vi "LIDAR V5 FPGA Main.vi"() -> ()   [LabVIEW 2015]
uses:
  <vilib>/Platform/TimedLoop/XDataNode/XDataNode.xnode
  <vilib>/Platform/TimedLoop/XDataNode/nitl_modes.ctl
  <vilib>/Platform/TimedLoop/XDataNode/XDNodeRunTimeDep.lvlib
  <vilib>/Platform/TimedLoop/XDataNode/wakeup.ctl
  <vilib>/Platform/TimedLoop/XDataNode/timing_clust.ctl
  <vilib>/eio/EIONode/EIONode.xnode
  <vilib>/rvi/eio/common/nirviEmuTemplateMethod_errors.vi
  <vilib>/rvi/DataTransferAndStorage/Container/XNode/niFpgaContainer.xnode
  <vilib>/rvi/FIFO/Fifo_Resource/nirvififoEmulationRead.vi
  LIDAR V2 Globals.vi
  <vilib>/rvi/Memory/Memory_Emulation/nirvimemoryFastEmulation.vi
  <vilib>/rvi/Memory/Memory_Emulation/nirvimemoryEmulation.vi
  Controls/FPGA Nain State.ctl
  Controls/Algorithm State.ctl
  <vilib>/rvi/interface/RandomDataEmulation/nirviRandomDataFpgaReadWriteTemplate.vi
panel:
  in  "y 6":u32
  in  "y 5":u32
  out "PulseIndex":i16
  in  "WaitForPulseEndDelay":u8=3
  in  "y":i16
  in  "y 2":i16
  in  "y 3":i16
  in  "y 4":i16
  out "EnableSignal":bool
  out "ActiveLedIndex":u16
  in  "EndOfPulseGen 2":bool
  in  "SamplingEnable":bool
  in  "SingleFrame":bool
  out "MainState":T1
  in  "NoOfLeds":u16=320
  in  "PulsePerLed":i16=199
  in  "FillDark":bool
  in  "DarkData":fxp<+/-,22,22>
  in  "DarkAdd":u32
  in  "SubstractDark":bool
  in  "FillVga":bool
  in  "VgaData":i16
  in  "VgaAdd":u32
  in  "ScanMode":bool
  in  "FrameStartDisable":bool=TRUE
  out "MeanTimeouts":u16
  in  "MaxStartSample":u32
  out "Port1":u8 format="%.0b"
  out "Port1Bit5":bool
  out "Port1Bit4":bool
  out "Port0":u8 format="%.0b"
  in  "PFI2":bool
  in  "PFI3":bool
  in  "ActiveLedIndexDeb":u16
  in  "LedScanDebEn":bool
  out "User Command Idle":bool
  out "User Command Status":u8
  out "User Error":bool
  out "Configured?":bool
  out "PLL Locked":bool
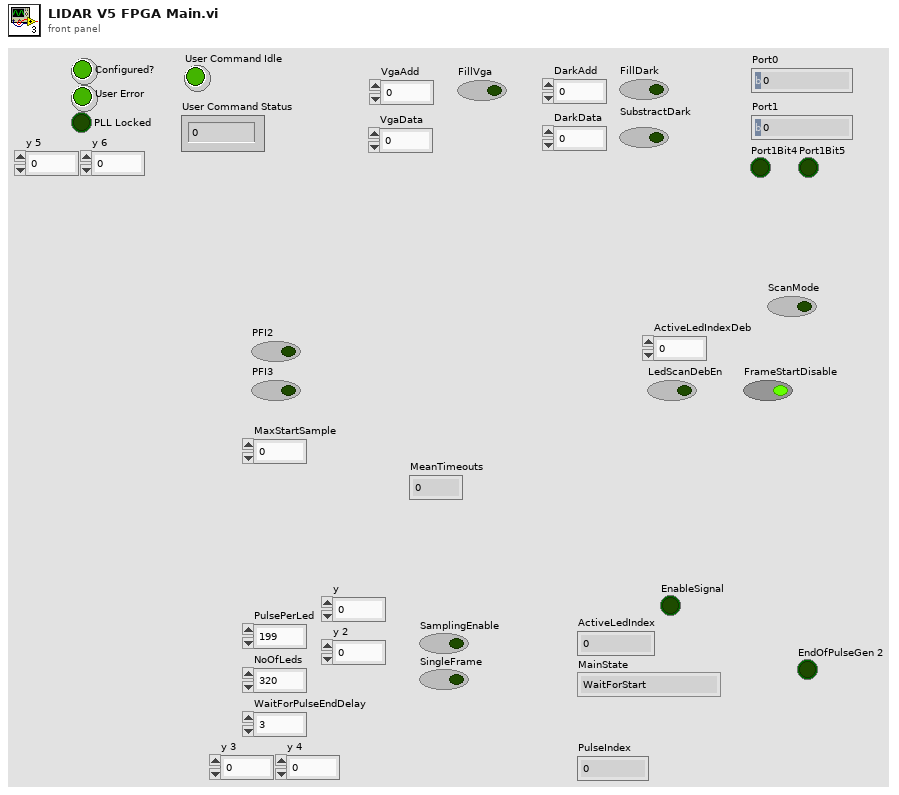
[diagram p1: front panel]
types:
  T1 = typedef "FPGA Nain State.ctl" = enum16{"WaitForStart", "SelectActiveLed", "WaitForNextPulse", "ActivatePulseCycle", "Error"}
  T2 = typedef "XDNodeRunTimeDep.lvlib/timing_clust.ctl" = cluster{"Expected End [f-1]":u64, "Actual End [f-1]":u64, "Finished Late? [f-1]":bool, "Expected End [i-1]":u64, "Actual End [i-1]":u64, "Finished Late? [i-1]":bool, "Expected Start [i]":u64, "Actual Start [i]":u64, "Expected Start [f]":u64, "Actual Start [f]":u64, "Source Name":string, "Structure Name":string, "Period":i64, "Deadline":i64, "Offset":i64, "Start":i64, "Priority":i32, "Timeout":i32, "Mode":T3, "Wakeup Reason":T4, "Error":errorcluster, "Source Type":string, "Secondary Source Type":string, "Global End Time":u64, "Global Start Time":u64, "Frame Duration":u64, "Iteration Duration":u64, "Assigned CPU":i32, "I/O Scan Engine Mode":u32}
  T3 = typedef "XDNodeRunTimeDep.lvlib/nitl_modes.ctl" = enum32{"No Change", "Process missed periods, maintain original phase", "Discard missed periods, maintain original phase", "Process missed periods, ignore original phase", "Discard missed periods, ignore original phase"}
  T4 = typedef "XDNodeRunTimeDep.lvlib/wakeup.ctl" = enum32{"Normal", "Aborted", "Asynchronous wakeup", "Timing source error", "Timed loop error", "Timeout"}
  T5 = typedef "Algorithm State.ctl" = enum16{"WaitForStart", "GetNextSignalElement", "WaitForNextSignalElem", "MultWithSinc", "CalcMax"}
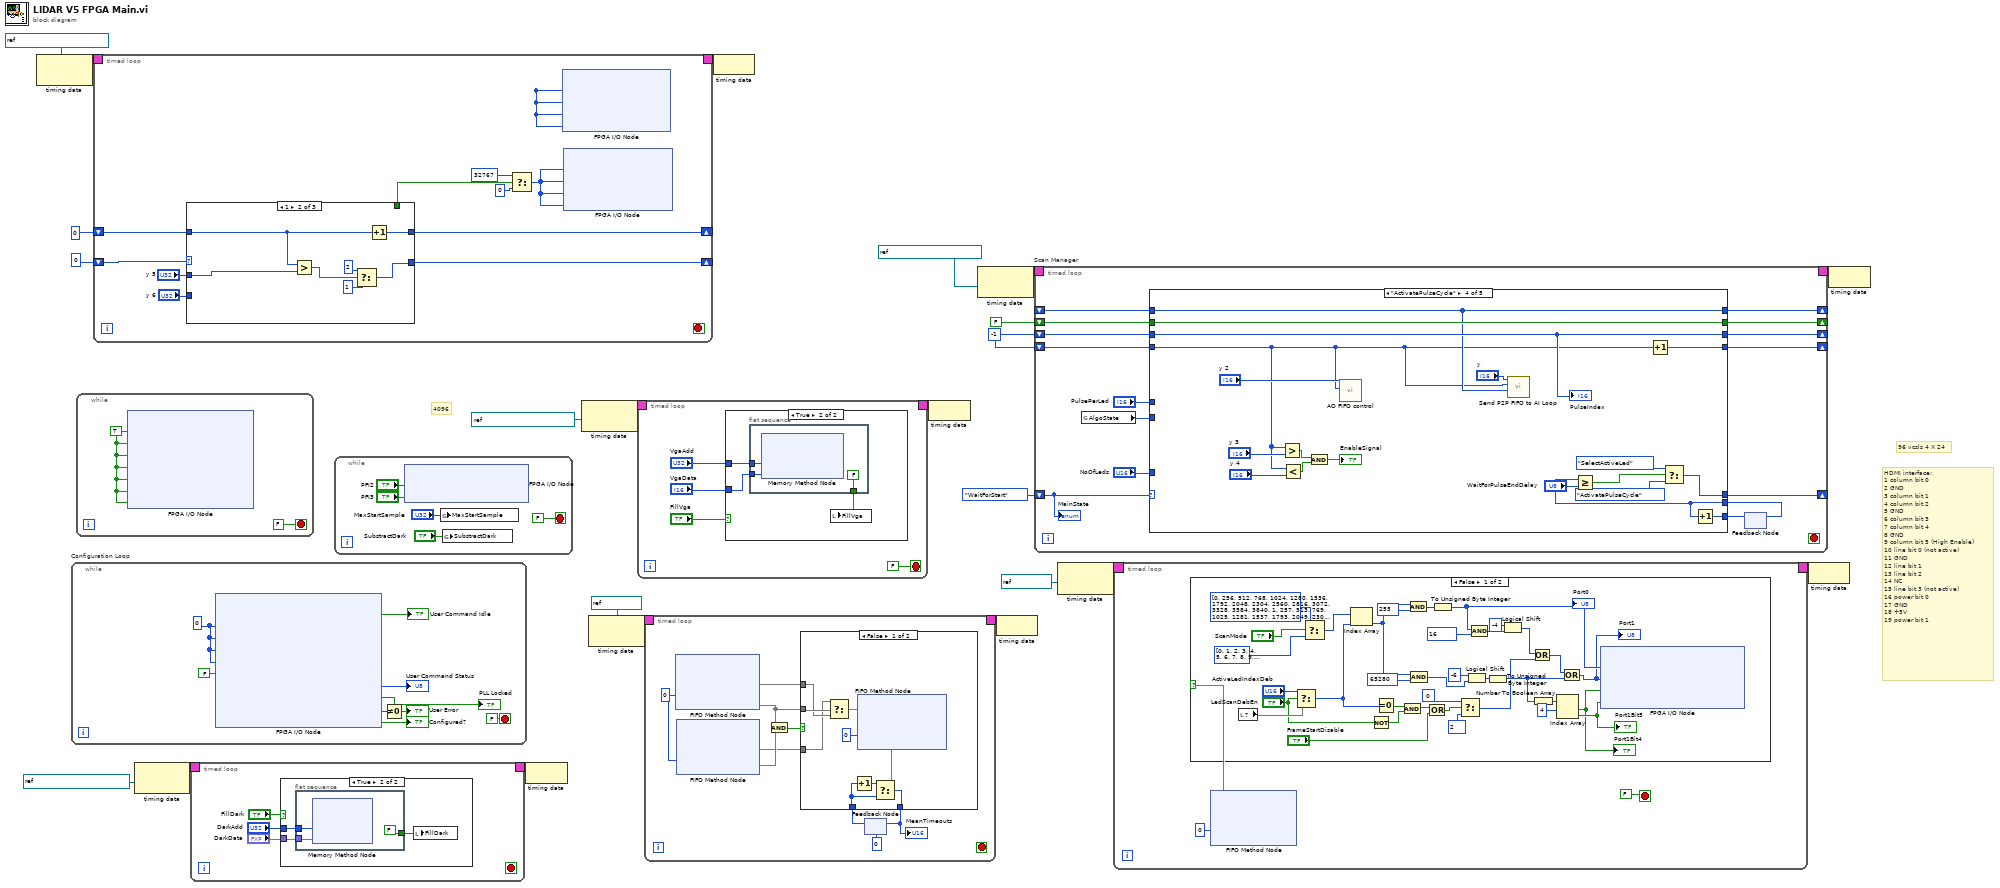
[diagram p0: block diagram]
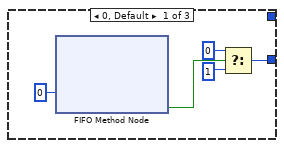
[diagram p2: hidden frame]
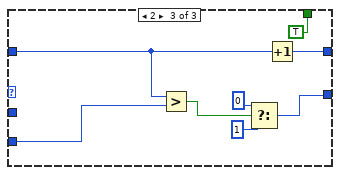
[diagram p3: hidden frame]
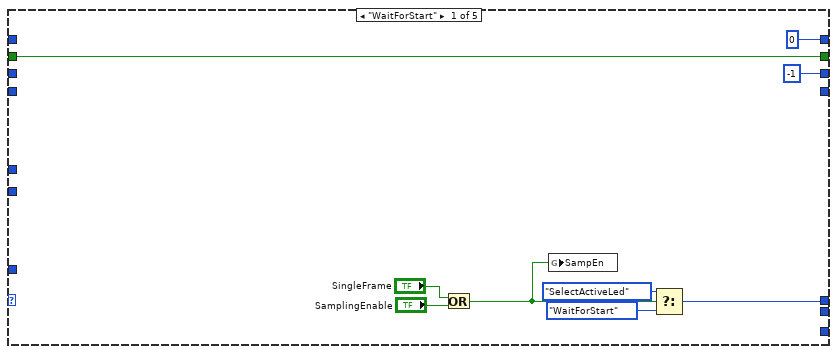
[diagram p4: hidden frame]
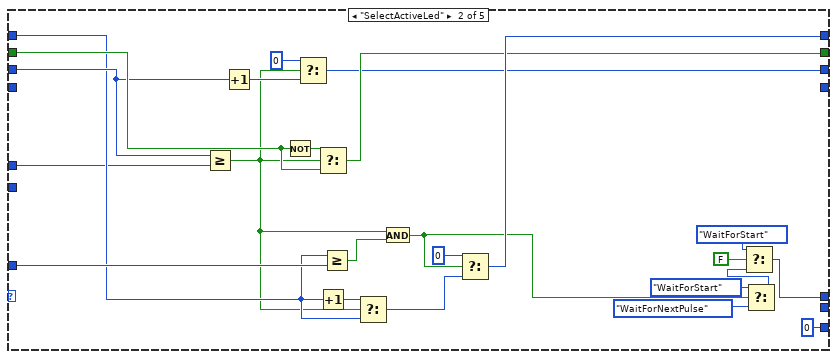
[diagram p5: hidden frame]
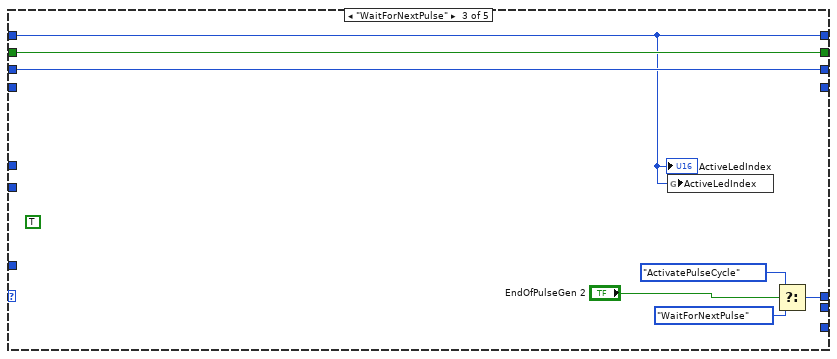
[diagram p6: hidden frame]
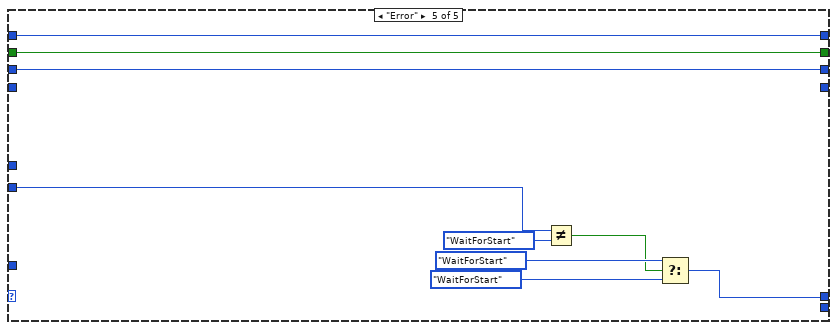
[diagram p7: hidden frame]
diagram:
  w6 = i16 -1
  # "HDMI interface:\n1 column bit 0\n2 GND\n3 column bit 1\n4 column bit 2\n5 GND\n6 column bit 3\n7 column bit 4 \n8 GND \n9 column bit 5 (High Enable) \n10 line bit 0 (not active) \n11 GND \n12 line bit 1 \n13 line bit 2 \n14 NC \n15 line bit 3 (not active) \n16 power bit 0 \n17 GND \n18 +5V \n19 power bit 1"
  # "96 vcsls 4 X 24"
  # "4096"
  n1 = node-c288(refnum<k21> "IO Module\\Data Clock" ("Source Name")) -> (w5:T2)
  n2 = while "Configuration Loop" {
    stop <- FALSE stop-if-true
    w25 = u8 0 ("SPI Device")
    n3 = xnode "FPGA I/O Node"("IO Module\\SPI Device"=w25, "IO Module\\User Command"=w25, "IO Module\\User Data 0"=w25, "IO Module\\User Data 1"=w25, "IO Module\\User Command Commit"=FALSE ("IO Module\\User Command Commit")) -> ("IO Module\\User Command Idle"=→"User Command Idle":bool, "IO Module\\User Command Status"=→"User Command Status":u8, "IO Module\\PLL Locked"=→"PLL Locked":bool, "IO Module\\User Error"=w29:u8, "IO Module\\Initialization Done"=→"Configured?":bool)  [unwired: 10 in, 10 out]
    n4 = Not Equal To 0?(x=w29) -> (x != 0?=→"User Error":bool)
  }
  n5 = while {
    stop <- FALSE stop-if-true
    w33 = TRUE ("IO Module\\DIO Port 0 WE")
    n6 = xnode "FPGA I/O Node"("IO Module\\DIO Port 0 WE"=w33, "IO Module\\DIO Port 1 WE"=w33, "IO Module\\PFI 0 WE"=w33, "IO Module\\PFI 1 WE"=w33, "IO Module\\PFI 2 WE"=w33, "IO Module\\PFI 3 WE"=w33, "IO Module\\AO Data Sync"=w33) -> ()  [unwired: 7 in, 7 out]
  }
  n7 = timed-loop {
    timing: w5 -> [_]
    timing-out: [_] -> w4
    shift-right: [w40] -> _
    shift-left: u8 0 -> [w41]
    shift-right: [w38] -> _
    shift-left: u32 0 -> [w39]
    stop <- _ stop-if-true
    n8 = case shown="1" w41 {
      tunnel: [w47 w52 w60] -> w40
      tunnel: w39 -> [_ w56 w63]
      tunnel: [_ w57 w65] -> w38
      tunnel: [_ _ TRUE] -> w37
      tunnel: "y 5" -> [_ w55 _]
      tunnel: "y 6" -> [_ _ w58]
      frame 0, Default {
        n9 = xnode ("FIFO Method Node")("Timeout"=0) -> ("Timed Out?"=w49:bool)  [unwired: 1 in, 2 out]
        n10 = Select(t=u8 0, s=w49, f=u8 1) -> (s? t:f=w47:u8)
      }
      frame 1 {
        n11 = Greater?(x=w56, y=w55) -> (0:w54:bool)
        n12 = Select(t=u8 2, s=w54, f=u8 1 ("t")) -> (s? t:f=w52:u8)
        n13 = Increment(x=w56) -> (x+1=w57:u32)
      }
      frame 2 {
        n14 = Greater?(x=w63, y=w58) -> (0:w62:bool)
        n15 = Select(t=u8 0, s=w62, f=u8 1 ("t")) -> (s? t:f=w60:u8)
        n16 = Increment(x=w63) -> (x+1=w65:u32)
      }
    }
    n17 = Select(t=i16 32767 ("IO Module\\AO 0 N"), s=w37, f=i16 0) -> (s? t:f=w44:i16)
    n18 = xnode "FPGA I/O Node"("IO Module\\AO 1 N-1"=w45, "IO Module\\AO 1 N-2"=w45, "IO Module\\AO 1 N-3"=w45) -> ("IO Module\\AO 1 N"=w45:i16)  [unwired: 4 in, 4 out]
    n19 = xnode "FPGA I/O Node"("IO Module\\AO 0 N-3"=w44, "IO Module\\AO 0 N-2"=w44, "IO Module\\AO 0 N-1"=w44, "IO Module\\AO 0 N"=w44) -> ()  [unwired: 4 in, 4 out]
  }
  n20 = node-c288(refnum<k21> "40 MHz Onboard Clock" ("Source Name")) -> (w14:T2)
  n21 = timed-loop {
    timing: w14 -> [_]
    timing-out: [_] -> w13
    stop <- _ stop-if-true
    n22 = case shown="True" "FillDark" {
      tunnel: "DarkAdd" -> [_ w73]
      tunnel: "DarkData" -> [_ w72]
      frame False {
      }
      frame True {
        n23 = flat-sequence {
          tunnel: w73 -> [w76]
          tunnel: w72 -> [w75]
          tunnel: [FALSE] -> w71
          frame #0 {
            n24 = xnode ("Memory Method Node")("Address"=w76, "Data"=w75) -> ()  [unwired: 1 in, 1 out]
          }
        }
        n25 = local write "FillDark"(w71) -> ()
      }
    }
  }
  n26 = while {
    stop <- FALSE stop-if-true
    n27 = xnode "FPGA I/O Node"("IO Module\\PFI 2 Wr Data"="PFI2", "IO Module\\PFI 3 Wr Data"="PFI3") -> ()  [unwired: 2 in, 2 out]
    n28 = global write "LIDAR V2 Globals.vi" "MaxStartSample"("MaxStartSample") -> ()
    n29 = global write "LIDAR V2 Globals.vi" "SubstractDark"("SubstractDark") -> ()
  }
  n30 = node-c288(w13) -> ()
  n31 = node-c288(refnum<k21> "IO Module\\Data Clock" ("Source Name")) -> (w17:T2)
  n32 = node-c288(refnum<k21> "130MHz" ("Source Name")) -> (w20:T2)
  n33 = timed-loop {
    timing: w17 -> [_]
    timing-out: [_] -> w16
    stop <- FALSE stop-if-true
    n34 = case shown="True" "FillVga" {
      tunnel: "VgaAdd" -> [_ w90]
      tunnel: "VgaData" -> [_ w89]
      frame False {
      }
      frame True {
        n35 = flat-sequence {
          tunnel: w90 -> [w93]
          tunnel: w89 -> [w92]
          tunnel: [FALSE ("FillVga")] -> w88
          frame #0 {
            n36 = xnode ("Memory Method Node")("Address"=w93, "Data"=w92) -> ()  [unwired: 1 in, 1 out]
          }
        }
        n37 = local write "FillVga"(w88) -> ()
      }
    }
  }
  n38 = timed-loop {
    timing: w20 -> [_]
    timing-out: [_] -> w19
    stop <- _ stop-if-true
    w104 = 0 ("Timeout")
    n39 = xnode ("FIFO Method Node")("Timeout"=w104) -> ("Element"=w100, "Timed Out?"=w101)  [unwired: 1 in, 1 out]
    n40 = xnode ("FIFO Method Node")("Timeout"=w104) -> ("Element"=w99, "Timed Out?"=w103)  [unwired: 1 in, 1 out]
    n41 = And(x=w101, y=w103) -> (x .and. y?=w102:bool)
    n42 = feedback #1(u16 0) -> (w97:u16)
    n43 = case shown="False" w102 {
      tunnel: w101 -> [w112 _]
      tunnel: w100 -> [w111 _]
      tunnel: w99 -> [w110 _]
      tunnel: w97 -> [w107 w114]
      tunnel: [w108 w114] -> w96
      frame False {
        n44 = Select(t=w110, s=w112, f=w111) -> (s? t:f=w109:dbl)
        n45 = Increment(x=w107) -> (x+1=w106:u16)
        n46 = xnode ("FIFO Method Node")("Element"=w109, "Timeout"=0) -> ("Timed Out?"=w105)  [unwired: 1 in, 1 out]
        n47 = Select(t=w106, s=w105, f=w107) -> (s? t:f=w108:u16)
      }
      frame True {
      }
    }
    "MeanTimeouts" <- w96
    n48 = feedback-in #1(w96) -> ()
  }
  n49 = node-c288(w4) -> ()
  n50 = node-c288(w16) -> ()
  n51 = node-c288(refnum<k21> "IO Module\\Data Clock" ("Source Name")) -> (w11:T2)
  n52 = node-c288(w19) -> ()
  n53 = timed-loop "Scan Manager" {
    timing: w11 -> [_]
    timing-out: [_] -> w10
    shift-right: [w130] -> _
    shift-left: FPGA_Nain_State."WaitForStart" ("MainState") -> [w131]
    shift-right: [w124] -> _
    shift-left: _ -> [w129]
    shift-right: [w126] -> _
    shift-left: FALSE -> [w128]
    shift-right: [w127] -> _
    shift-left: w6 -> [w125]
    shift-right: [w117] -> _
    shift-left: w6 -> [w118]
    stop <- _ stop-if-true
    n54 = global read "LIDAR V2 Globals.vi" "AlgoState"() -> (w123:T5)
    n55 = feedback #2() -> (w120:u8)  [unwired: 1 in]
    n56 = case shown="\"ActivatePulseCycle\"" w131 {
      tunnel: [w138 w161 w167 w183 w194] -> w130
      tunnel: [u16 0 ("ActiveLedIndex") w157 w166 w179 w199] -> w124
      tunnel: w129 -> [_ w149 w166 w179 w199]
      tunnel: [w135 w156 w171 w182 w198] -> w126
      tunnel: w128 -> [w135 w159 w171 w182 w198]
      tunnel: [i16 -1 ("t") w152 w170 w190 w197] -> w127
      tunnel: w125 -> [_ w155 w170 w190 w197]
      tunnel: w123 -> [_ _ _ _ w191]
      tunnel: "NoOfLeds" -> [_ w151 _ _ _]
      tunnel: [_ u8 0 _ w189 _] -> w121
      tunnel: w120 -> [_ _ _ w188 _]
      tunnel: "PulsePerLed" -> [_ w141 _ _ _]
      tunnel: w118 -> [_ _ _ w176 _]
      tunnel: [_ _ _ w181 _] -> w117
      frame "WaitForStart" {
        n57 = Or(x="SingleFrame", y="SamplingEnable") -> (x .or. y?=w132:bool)
        n58 = global write "LIDAR V2 Globals.vi" "SampEn"(w132) -> ()
        n59 = Select(t=FPGA_Nain_State."SelectActiveLed" ("MainState"), s=w132, f=FPGA_Nain_State."WaitForStart" ("MainState")) -> (s? t:f=w138:T1)
      }
      frame "SelectActiveLed" {
        n60 = Greater Or Equal?(x=w155, y=w141) -> (x >= y?=w144:bool)
        n61 = Increment(x=w155) -> (x+1=w154:i16)
        n62 = Not(x=w159) -> (.not. x?=w158:bool)
        n63 = Select(t=i16 0, s=w144, f=w154) -> (s? t:f=w152:i16)
        n64 = Select(t=w158, s=w144, f=w159) -> (s? t:f=w156:bool)
        n65 = Increment(x=w149) -> (x+1=w147:u16)
        n66 = Greater Or Equal?(x=w149, y=w151) -> (x >= y?=w145:bool)
        n67 = Select(t=w147, s=w144, f=w149) -> (s? t:f=w148:u16)
        n68 = And(x=w144, y=w145) -> (x .and. y?=w143:bool)
        n69 = Select(t=u16 0, s=w143, f=w148) -> (s? t:f=w157:u16)
        n70 = Select(t=FPGA_Nain_State."WaitForStart" ("MainState"), s=w143, f=FPGA_Nain_State."WaitForNextPulse" ("MainState")) -> (s? t:f=w162:T1)
        n71 = Select(t=FPGA_Nain_State."WaitForStart" ("MainState"), s=FALSE, f=w162) -> (s? t:f=w161:T1)
      }
      frame "WaitForNextPulse" {
        (unwired) TRUE
        n72 = global write "LIDAR V2 Globals.vi" "ActiveLedIndex"(w166) -> ()
        n73 = Select(t=FPGA_Nain_State."ActivatePulseCycle" ("MainState"), s="EndOfPulseGen 2", f=FPGA_Nain_State."WaitForNextPulse" ("MainState")) -> (s? t:f=w167:T1)
        "ActiveLedIndex" <- w166
      }
      frame "ActivatePulseCycle" {
        n74 = Greater?(x=w176, y="y 3") -> (0:w173:bool)
        n75 = Less?(x=w176, y="y 4") -> (x < y?=w174:bool)
        n76 = And(x=w173, y=w174) -> (x .and. y?=→"EnableSignal":bool)
        n77 = call "AO FIFO control.vi"("Counter"=w176, "StartPulse"="y 2") -> ()  [unwired: 10 in]
        n78 = call "Send P2P FIFO to AI Loop.vi"("ActiveLedIndex"=w179, "TimingCounter"=w176, "StartAcq"="y") -> ()  [unwired: 9 in]
        n79 = Greater Or Equal?(x=w188, y="WaitForPulseEndDelay") -> (x >= y?=w186:bool)
        n80 = Increment(x=w176) -> (x+1=w181:i16)
        n81 = Select(t=FPGA_Nain_State."SelectActiveLed" ("MainState"), s=w186, f=FPGA_Nain_State."ActivatePulseCycle" ("MainState")) -> (s? t:f=w183:T1)
        n82 = Increment(x=w188) -> (x+1=w189:u8)
        "PulseIndex" <- w190
      }
      frame "Error" {
        n83 = Not Equal?(x=w191, y=Algorithm_State."WaitForStart") -> (x != y?=w192:bool)
        n84 = Select(t=FPGA_Nain_State."WaitForStart", s=w192, f=FPGA_Nain_State."WaitForStart" ("MainState")) -> (s? t:f=w194:T1)
      }
    }
    n85 = feedback-in #2(w121) -> ()
    "MainState" <- w131
  }
  n86 = node-c288(refnum<k21> "130MHz" ("Source Name")) -> (w23:T2)
  n87 = timed-loop {
    timing: w23 -> [_]
    timing-out: [_] -> w22
    stop <- FALSE stop-if-true
    n88 = xnode ("FIFO Method Node")("Timeout"=0) -> ("Timed Out?"=w202)  [unwired: 1 in, 2 out]
    n89 = case shown="False" w202 {
      frame False {
        n90 = local read item#-1() -> (w235)
        n91 = Select(t="ActiveLedIndexDeb", s="LedScanDebEn", f=w235) -> (s? t:f=w220:u16)
        n92 = Select(t=u16[] [0, 256, 512, 768, 1024, 1280, 1536, 1792, 2048, 2304, 2560, 2816, 3072, 3328, 3584, 3840, 1, 257, 513, 769, 1025, 1281, 1537, 1793, 2049, 2305, 2561, 2817, 3073, 3329, 3585, 3841, 2, 258, 514, 770, 1026, 1282, 1538, 1794, 2050, 2306, 2562, 2818, 3074, 3330, 3586, 3842, 3, 259, 515, 771, 1027, 1283, 1539, 1795, 2051, 2307, 2563, 2819, 3075, 3331, 3587, 3843, 4, 260, 516, 772, 1028, 1284, 1540, 1796, 2052, 2308, 2564, 2820, 3076, 3332, 3588, 3844, 5, 261, 517, 773, 1029, 1285, 1541, 1797, 2053, 2309, 2565, 2821, 3077, 3333, 3589, 3845, 6, 262, 518, 774, 1030, 1286, 1542, 1798, 2054, 2310, 2566, 2822, 3078, 3334, 3590, 3846, 7, 263, 519, 775, 1031, 1287, 1543, 1799, 2055, 2311, 2567, 2823, 3079, 3335, 3591, 3847, 8, 264, 520, 776, 1032, 1288, 1544, 1800, 2056, 2312, 2568, 2824, 3080, 3336, 3592, 3848, 9, 265, 521, 777, 1033, 1289, 1545, 1801, 2057, 2313, 2569, 2825, 3081, 3337, 3593, 3849, 10, 266, 522, 778, 1034, 1290, 1546, 1802, 2058, 2314, 2570, 2826, 3082, 3338, 3594, 3850, 11, 267, 523, 779, 1035, 1291, 1547, 1803, 2059, 2315, 2571, 2827, 3083, 3339, 3595, 3851, 12, 268, 524, 780, 1036, 1292, 1548, 1804, 2060, 2316, 2572, 2828, 3084, 3340, 3596, 3852, 13, 269, 525, 781, 1037, 1293, 1549, 1805, 2061, 2317, 2573, 2829, 3085, 3341, 3597, 3853, 14, 270, 526, 782, 1038, 1294, 1550, 1806, 2062, 2318, 2574, 2830, 3086, 3342, 3598, 3854, 15, 271, 527, 783, 1039, 1295, 1551, 1807, 2063, 2319, 2575, 2831, 3087, 3343, 3599, 3855, 16, 272, 528, 784, 1040, 1296, 1552, 1808, 2064, 2320, 2576, 2832, 3088, 3344, 3600, 3856, 17, 273, 529, 785, 1041, 1297, 1553, 1809, 2065, 2321, 2577, 2833, 3089, 3345, 3601, 3857, 18, 274, 530, 786, 1042, 1298, 1554, 1810, 2066, 2322, 2578, 2834, 3090, 3346, 3602, 3858, 19, 275, 531, 787, 1043, 1299, 1555, 1811, 2067, 2323, 2579, 2835, 3091, 3347, 3603, 3859] ("Array"), s="ScanMode", f=u16[] [0, 1, 2, 3, 4, 5, 6, 7, 8, 9, 10, 11, 12, 13, 14, 15, 16, 17, 18, 19, 256, 257, 258, 259, 260, 261, 262, 263, 264, 265, 266, 267, 268, 269, 270, 271, 272, 273, 274, 275, 512, 513, 514, 515, 516, 517, 518, 519, 520, 521, 522, 523, 524, 525, 526, 527, 528, 529, 530, 531, 768, 769, 770, 771, 772, 773, 774, 775, 776, 777, 778, 779, 780, 781, 782, 783, 784, 785, 786, 787, 1024, 1025, 1026, 1027, 1028, 1029, 1030, 1031, 1032, 1033, 1034, 1035, 1036, 1037, 1038, 1039, 1040, 1041, 1042, 1043, 1280, 1281, 1282, 1283, 1284, 1285, 1286, 1287, 1288, 1289, 1290, 1291, 1292, 1293, 1294, 1295, 1296, 1297, 1298, 1299, 1536, 1537, 1538, 1539, 1540, 1541, 1542, 1543, 1544, 1545, 1546, 1547, 1548, 1549, 1550, 1551, 1552, 1553, 1554, 1555, 1792, 1793, 1794, 1795, 1796, 1797, 1798, 1799, 1800, 1801, 1802, 1803, 1804, 1805, 1806, 1807, 1808, 1809, 1810, 1811, 2048, 2049, 2050, 2051, 2052, 2053, 2054, 2055, 2056, 2057, 2058, 2059, 2060, 2061, 2062, 2063, 2064, 2065, 2066, 2067, 2304, 2305, 2306, 2307, 2308, 2309, 2310, 2311, 2312, 2313, 2314, 2315, 2316, 2317, 2318, 2319, 2320, 2321, 2322, 2323, 2560, 2561, 2562, 2563, 2564, 2565, 2566, 2567, 2568, 2569, 2570, 2571, 2572, 2573, 2574, 2575, 2576, 2577, 2578, 2579, 2816, 2817, 2818, 2819, 2820, 2821, 2822, 2823, 2824, 2825, 2826, 2827, 2828, 2829, 2830, 2831, 2832, 2833, 2834, 2835, 3072, 3073, 3074, 3075, 3076, 3077, 3078, 3079, 3080, 3081, 3082, 3083, 3084, 3085, 3086, 3087, 3088, 3089, 3090, 3091, 3328, 3329, 3330, 3331, 3332, 3333, 3334, 3335, 3336, 3337, 3338, 3339, 3340, 3341, 3342, 3343, 3344, 3345, 3346, 3347, 3584, 3585, 3586, 3587, 3588, 3589, 3590, 3591, 3592, 3593, 3594, 3595, 3596, 3597, 3598, 3599, 3600, 3601, 3602, 3603, 3840, 3841, 3842, 3843, 3844, 3845, 3846, 3847, 3848, 3849, 3850, 3851, 3852, 3853, 3854, 3855, 3856, 3857, 3858, 3859] ("Array")) -> (s? t:f=w206:u16[])
        n93 = Index Array(array=w206, index=w220) -> (element=w232:u16)
        n94 = Not(x="LedScanDebEn") -> (.not. x?=w217:bool)
        n95 = Equal To 0?(x=w220) -> (x = 0?=w219:bool)
        n96 = And(x=w219, y=w217) -> (x .and. y?=w215:bool)
        n97 = And(x=w232, y=u16 255) -> (x .and. y?=w230:u16)
        n98 = And(x=w232, y=u16 65280) -> (x .and. y?=w229:u16)
        n99 = Or(x=w215, y="FrameStartDisable") -> (x .or. y?=w210:bool)
        n100 = To Unsigned Byte Integer(number=w230) -> (unsigned 8bit integer=w226:u8)
        "Port0" <- w226
        n101 = Select(t=u8 0, s=w210, f=u8 2) -> (s? t:f=w212:u8)
        n102 = Logical Shift(y=i16 -6, x=w229) -> (x << y=w228:u16)
        n103 = And(x=w226, y=u8 16) -> (x .and. y?=w225:u8)
        n104 = To Unsigned Byte Integer(number=w228) -> (unsigned 8bit integer=w222:u8)
        n105 = Logical Shift(y=i16 -4, x=w225) -> (x << y=w216:u8)
        n106 = Or(x=w216, y=w212) -> (x .or. y?=w211:u8)
        n107 = Number To Boolean Array(number=w222) -> (Boolean array=w239:bool[])
        n108 = Index Array(array=w239, index #1=4 ("index")) -> (element #1=w223:bool, element #2=w237:bool)  [unwired: 1 in]
        "Port1Bit4" <- w223
        "Port1Bit5" <- w237
        n109 = Or(x=w211, y=w222) -> (x .or. y?=w221:u8)
        "Port1" <- w221
        n110 = xnode "FPGA I/O Node"("IO Module\\DIO Port 0 Wr Data"=w226, "IO Module\\DIO Port 1 Wr Data"=w221, "IO Module\\PFI 0 Wr Data"=w223, "IO Module\\PFI 1 Wr Data"=w237) -> ()  [unwired: 4 in, 4 out]
      }
      frame True {
      }
    }
  }
  n111 = node-c288(w22) -> ()
  n112 = node-c288(w10) -> ()
